vi "Calculate number of 1's in a Binary Number.vi"(11 "BINARY NUMBER":i32 format="%b") -> (3 "Number of 1's":i32)   [LabVIEW 2020]
doc: "This VI will calculate Number of 1's in a Binary Number."
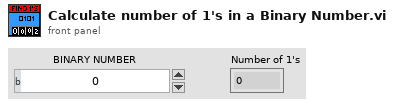
[diagram p1: front panel]
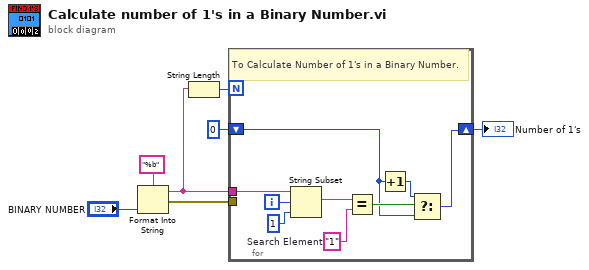
[diagram p0: block diagram]
diagram:
  n1 = Format Into String(format string="%b", "BINARY NUMBER") -> (resulting string=w3:string, error out=w5:errorcluster)  [unwired: 2 in]
  n2 = String Length(string=w3) -> (length=w4:i32)
  n3 = for {
    N: w4 -> [_]
    tunnel: w3 -> [w16]
    tunnel: w5 -> [_]
    shift-right: [w8] -> w1
    shift-left: 0 ("length (rest)") -> [w9]
    i -> [w15]
    w12 = "1"  # Search Element
    # "To Calculate Number of 1's in a Binary Number."
    n4 = String Subset(string=w16, offset (0)=w15, length (rest)=1 ("length (rest)")) -> (substring=w13:string)
    n5 = Equal?(x=w13, y=w12) -> (x = y?=w11:bool)
    n6 = Increment(x=w9) -> (x+1=w10:i32)
    n7 = Select(t=w10, s=w11, f=w9) -> (s? t:f=w8:i32)
  }
  "Number of 1's" <- w1
